vi "niScope Get Session Reference.vi"(0 "instrument handle":refnum<k15>, 11 "error in":errorcluster) -> (4 "instrument handle out":refnum<k15>, 6 "session reference":refnum<k20>, 15 "error out":errorcluster)   [LabVIEW 2013]
doc: "Extracts a session that can be passed to NI-TClk VIs. Session References are of generic type, which means that the corresponding wires are blue-green, unlike the wires for regular instrument driver sessions."
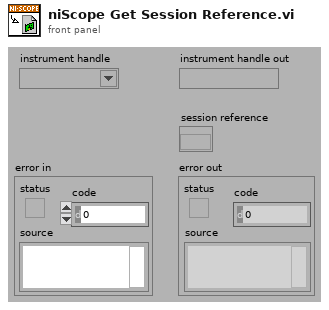
[diagram p1: front panel]
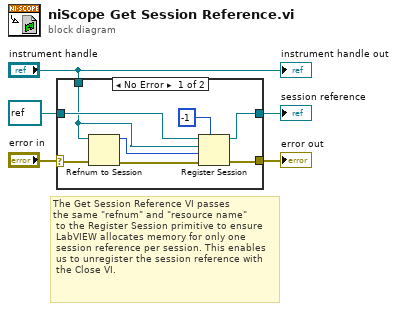
[diagram p0: block diagram]
diagram:
  # "The Get Session Reference VI passes \nthe same \"refnum\" and \"resource name\"\n to the Register Session primitive to ensure\n LabVIEW allocates memory for only one\n session reference per session. This enables\n us to unregister the session reference with\n the Close VI."
  n1 = case shown="No Error" "error in" {
    selector: "error in" -> [w10 w15]
    tunnel: [w11 w15] -> w5
    tunnel: "instrument handle" -> [w6 _]
    tunnel: [w12 w14] -> w2
    tunnel: refnum<k20> refnum ("session reference") -> [w7 w14]
    frame No Error {
      n2 = Refnum to Session(4:w10, 7:w6) -> (0:w9:errorcluster, 3:w8:u64)
      n3 = Register Session(7:-1 ("cleanup mode (default to class = 0)"), 8:w9, 9:w8, 10:w6, 11:w7) -> (0:w11:errorcluster, 3:w12:refnum<k20>)
    }
    frame Error {
    }
  }
  "error out" <- w5
  "session reference" <- w2
  "instrument handle out" <- "instrument handle"
